vi "Initialise.vi"(8 "error in (no error)":errorcluster, 10 "Initial Config":T1={"Log Files Directory"=path "", "Max Lines Per File"=10000}, 11 "Process":refnum<vi>) -> (0 "error out":errorcluster, 3 "Actor out":refnum<class "Logger Actor.lvclass">, 5 "Mailboxes":cluster{"Mailbox":refnum<event-registration>})   [LabVIEW 2020, in "RTAF.lvlib" / "Logger Actor.lvclass"]
uses:
  Logger Actor.lvclass
  C:/dev/PGS/2001 - TBCM/Source/RT/RTAF/Source/RTAF/Actors/Base Actor/Actor/Actor.lvclass
  Base Actor/Actor/Message.ctl
  Config.ctl
  API/Logger Actor API.lvclass
  C:/dev/PGS/2001 - TBCM/Source/RT/RTAF/Source/RTAF/Actors/Base Actor/API/Actor API.lvclass
  Log/Log.lvclass
  Logger Actor.lvclass/Logger Actor.ctl
  Global References.vi
  Base Actor/API/Actor API.lvclass
  RTAF.lvlib
  Base Actor/Actor/Actor.lvclass
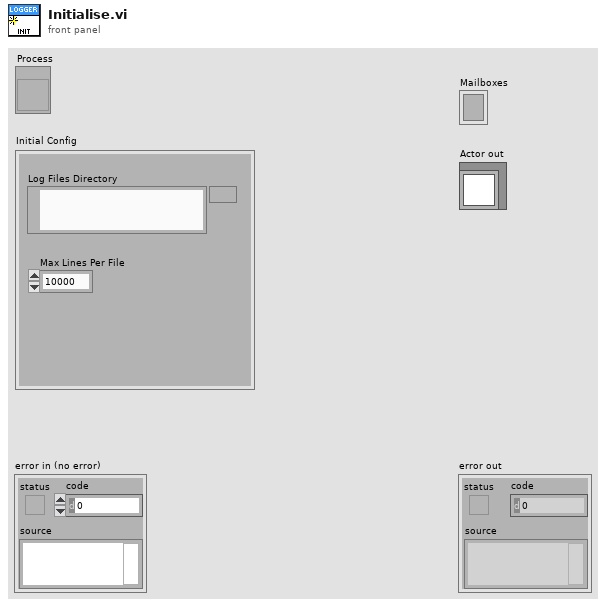
[diagram p1: front panel]
types:
  T1 = typedef "RTAF.lvlib/Logger Actor.lvclass/Config.ctl" = cluster{"Log Files Directory":path, "Max Lines Per File":i32}
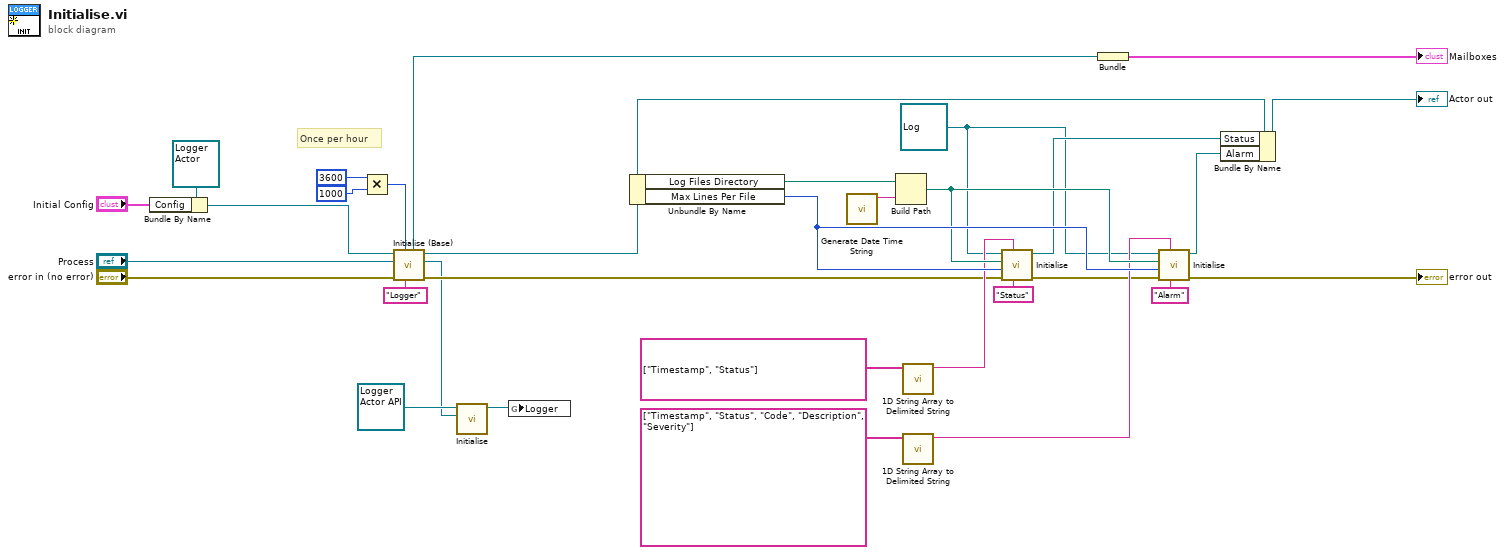
[diagram p0: block diagram]
diagram:
  w14 = refnum<class "Log.lvclass"> refnum ("Log in")
  # "Once per hour"
  n1 = Bundle By Name(cluster=refnum<class "Logger Actor.lvclass"> refnum ("Test Actor.lvclass"), "Config"="Initial Config") -> (w29:refnum<class "Logger Actor.lvclass">)
  n2 = Multiply(x=3600 ("Tick Period [100 ms]"), y=1000) -> (x*y=w26:i32)
  n3 = call "Initialise (Base).vi"("Name"="Logger", "Tick Period [100 ms]"=w26, "error in (no error)"="error in (no error)", "Process"="Process", "Actor in"=w29) -> ("error out"=w5:errorcluster, "Message Channel"=w3:refnum<user-event>, "Actor out"=w4:refnum<class "Logger Actor.lvclass">, "Mailbox"=w2:refnum<event-registration>)  [unwired: 3 in]
  n4 = call "Initialise.vi"("Message Channel"=w3, "Actor API in"=refnum<class "Logger Actor API.lvclass"> refnum ("Logger Actor API.lvclass")) -> ("Actor API out"=w1:refnum<class "Logger Actor API.lvclass">)  [unwired: 9 in]
  n5 = global write "Global References.vi" "Logger"(w1) -> ()
  n6 = Unbundle By Name(w4) -> ("Log Files Directory"=w22:path, "Max Lines Per File"=w24:i32)
  n7 = call "Generate Date Time String.vi"() -> ("Date time string"=w25:string)  [unwired: 10 in, 1 out]
  n8 = Build Path(base path=w22, name or relative path=w25) -> (appended path=w23:path)
  n9 = call <vilib>:"1D String Array to Delimited String.vi"("string array"=string[] ["Timestamp", "Status"]) -> ("delimited string"=w19:string)  [unwired: 10 in]
  n10 = call <vilib>:"1D String Array to Delimited String.vi"("string array"=string[] ["Timestamp", "Status", "Code", "Description", "Severity"]) -> ("delimited string"=w21:string)  [unwired: 10 in]
  n11 = call "Initialise.vi"("Filename"="Status", "Header"=w19, "error in (no error)"=w5, "Max Records"=w24, "Directory"=w23, "Log in"=w14) -> ("error out"=w17:errorcluster, "Log out"=w15:refnum<class "Log.lvclass">)  [unwired: 4 in]
  n12 = Bundle("Mailbox"=w2) -> (→"Mailboxes":cluster{"Mailbox":refnum<event-registration>})  [unwired: 1 in]
  n13 = call "Initialise.vi"("Filename"="Alarm", "Header"=w21, "error in (no error)"=w17, "Max Records"=w24, "Directory"=w23, "Log in"=w14) -> ("error out"=→"error out":errorcluster, "Log out"=w16:refnum<class "Log.lvclass">)  [unwired: 4 in]
  n14 = Bundle By Name(cluster=w4, "Status"=w15, "Alarm"=w16) -> (→"Actor out":refnum<class "Logger Actor.lvclass">)
